vi "configure.vi"(8 "error in (no error)":errorcluster, 11 "DL090628DSSTraceProcessor in":refnum<class "TraceProcessorDL090628DSS.lvclass">) -> (0 "error out":errorcluster, 3 "DL090628DSSTraceProcessor out":refnum<class "TraceProcessorDL090628DSS.lvclass">)   [LabVIEW 2010, in "TraceProcessorDL090628DSS.lvclass"]
doc: "The dynamic dispatch version of this VI loads and displays the configuration file associated with the plug-in object. The user modify and save the configuration data."
uses:
  TraceProcessorDL090628DSS.lvclass
  TraceProcessorDL090628DSS.lvclass/TraceProcessorDL090628DSS.ctl
  common/classes/GenericComponent/GenericComponent/GenericComponent.lvclass
panel:
  in  "Tab Control":enum32{"Description", "Configuration settings"}(tab)
  in  "number of baseline sampling points":i32
  out "Configuration":string
  in  "cancel button":bool
  in  "save button":bool
  # "Configure TraceProcessorDL090628DSS"
  # "The TraceProcessorDL090628DSS calculates the dS/S (\"delta S over S\") of a signal intensity trace."
  # "The number of intensity values used to calculate \"S0\" at the beginning of a trace (in order to calculate \"(S-S0)/S0\")."
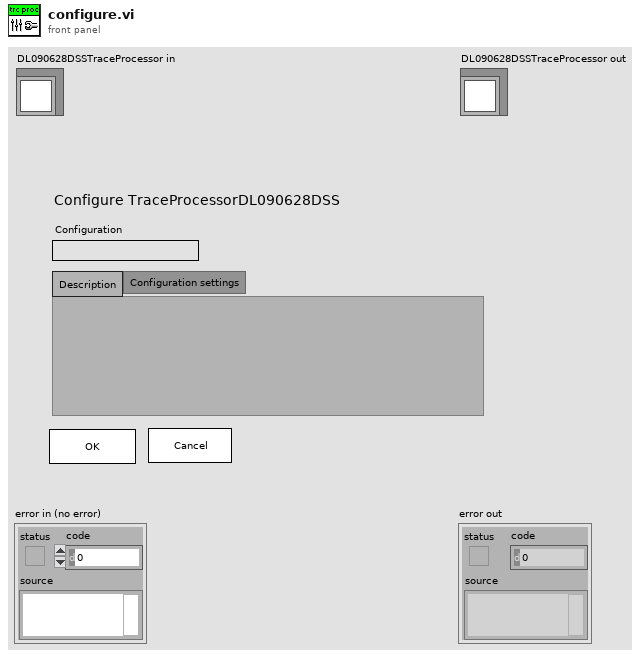
[diagram p1: front panel]
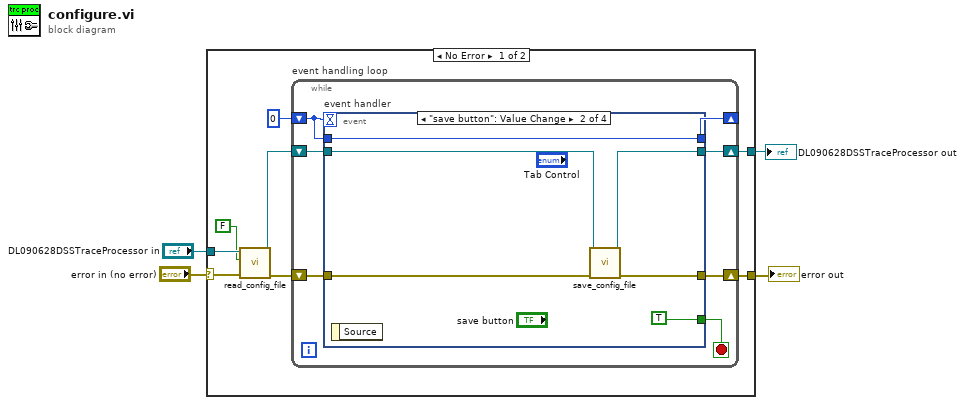
[diagram p0: block diagram]
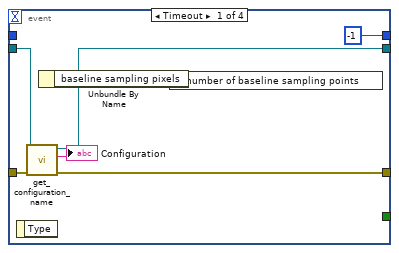
[diagram p2: hidden frame]
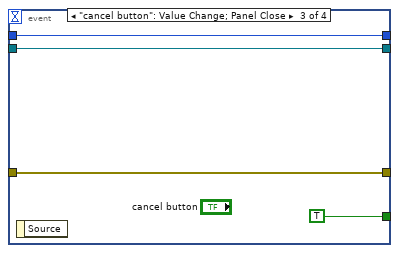
[diagram p3: hidden frame]
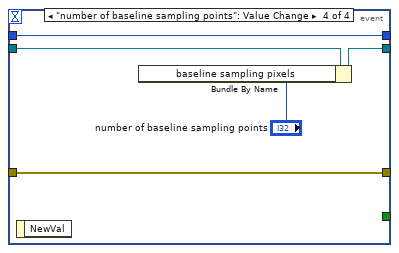
[diagram p4: hidden frame]
diagram:
  n1 = case shown="No Error" "error in (no error)" {
    selector: "error in (no error)" -> [w12 w43]
    tunnel: [w10 w43] -> w3
    tunnel: "DL090628DSSTraceProcessor in" -> [w9 w42]
    tunnel: [w5 w42] -> w1
    frame No Error {
      n2 = call-dynamic "read_config_file.vi"("error in (no error)"=w12, "force load?"=FALSE, "GenericPlugin in"=w9) -> ("error out"=w11:errorcluster, "GenericPlugin out"=w7:refnum<class "TraceProcessorDL090628DSS.lvclass">)  [unwired: 7 out]
      n3 = while "event handling loop" {
        shift-right: [w18] -> w10
        shift-left: w11 -> [w19]
        shift-right: [w15] -> w5
        shift-left: w7 -> [w17]
        shift-right: [w14] -> _
        shift-left: 0 -> [w16]
        stop <- w13 stop-if-true
        n4 = event "event handler" shown="[1] \"save button\": Value Change" {
          selector: _ -> [_ _ _ _]
          dyn-events: _ -> [_ _ _ _]
          timeout: w16 -> [_ _ _ _]
          tunnel: w19 -> [w24 w31 w36 w40]
          tunnel: [w21 w30 w36 w40] -> w18
          tunnel: w17 -> [w23 w27 w34 w38]
          tunnel: w16 -> [_ w32 w35 w41]
          tunnel: [-1 w32 w35 w41] -> w14
          tunnel: [w22 w29 w34 w37] -> w15
          tunnel: [_ TRUE TRUE _] -> w13
          event Timeout {
            n5 = event-data() -> ()  [unwired: 2 out]
            n6 = call "get_configuration_name.vi"("error in (no error)"=w24, "GenericPlugin.lvclass in"=w23) -> ("error out"=w21:errorcluster, "configuration name"=→"Configuration":string, "GenericPlugin.lvclass out"=w22:refnum<class "TraceProcessorDL090628DSS.lvclass">)  [unwired: 7 in]
            n7 = Unbundle By Name(w22) -> ("baseline sampling pixels"=w26:i32)
            n8 = local write "number of baseline sampling points"(w26) -> ()
          }
          event "save button": Value Change {
            n9 = event-data() -> ()  [unwired: 2 out]
            n10 = call-dynamic "save_config_file.vi"("error in (no error)"=w31, "GenericPlugin in"=w27) -> ("error out"=w30:errorcluster, "GenericPlugin out"=w29:refnum<class "TraceProcessorDL090628DSS.lvclass">)  [unwired: 1 in, 7 out]
          }
          event "cancel button": Value Change; Panel Close {
            n11 = event-data() -> ()  [unwired: 2 out]
          }
          event "number of baseline sampling points": Value Change {
            n12 = event-data() -> ()  [unwired: 2 out]
            n13 = Bundle By Name(cluster=w38, "baseline sampling pixels"="number of baseline sampling points") -> (w37:refnum<class "TraceProcessorDL090628DSS.lvclass">)
          }
        }
      }
    }
    frame Error {
    }
  }
  "error out" <- w3
  "DL090628DSSTraceProcessor out" <- w1
